vi "CHD_RATE_CALC.vi"(9 "Time":dbl, 11 "Input":dbl) -> (3 "Output":dbl)   [LabVIEW 2019]
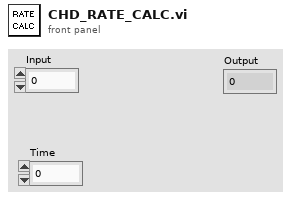
[diagram p1: front panel]
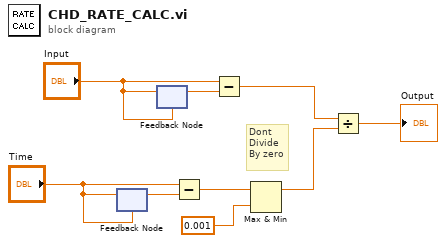
[diagram p0: block diagram]
diagram:
  # "Dont\nDivide \nBy zero"
  n1 = feedback #1("Time") -> (w5:dbl)
  n2 = feedback-in #1("Time") -> ()
  n3 = feedback #2("Input") -> (w7:dbl)
  n4 = feedback-in #2("Input") -> ()
  n5 = Subtract(x="Time", y=w5) -> (x-y=w1:dbl)
  n6 = Subtract(x="Input", y=w7) -> (x-y=w6:dbl)
  n7 = Max & Min(x=w1, y=0.001) -> (max(x,y)=w8:dbl)  [unwired: 1 out]
  n8 = Divide(x=w6, y=w8) -> (x/y=→"Output":dbl)
